vi "Get Installation Software Set.vi"(8 "error in (no error)":errorcluster, 11 "config session in":refnum<k21> caption="session in") -> (0 "error out":errorcluster, 1 "add-ons":T1[](array[typedef]) {"component type" items=["standard", "hidden", "system", "unknown", "startup"]}, 2 "software set":T1 {"component type" items=["standard", "hidden", "system", "unknown", "startup"]}, 3 "config session out":refnum<k21> caption="session out")   [LabVIEW 2013]
uses:
  <vilib>/nisyscfg/Software 1.2.ctl
  <vilib>/nisyscfg/Component Type.ctl
  <vilib>/nisyscfg/Get Available Sets.vi
  globals/Globals.vi
  <vilib>/nisyscfg/nisyscfg.lvlib
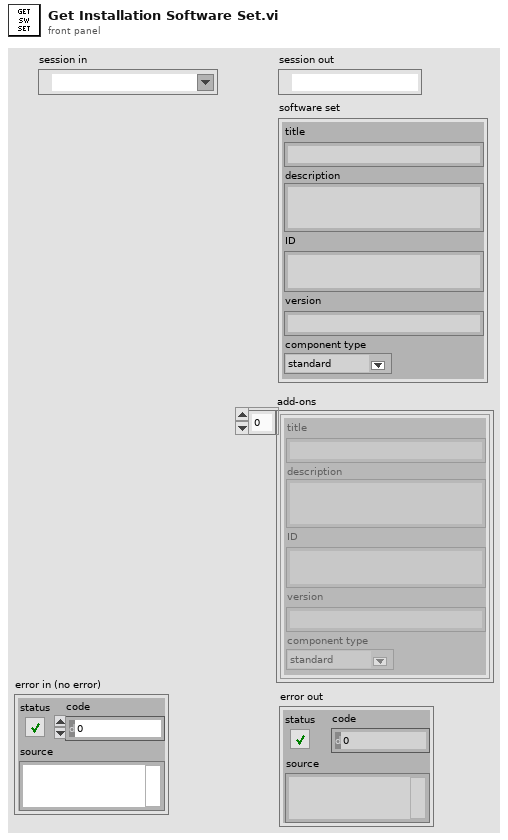
[diagram p1: front panel]
types:
  T1 = typedef "nisyscfg.lvlib/Software 1.2.ctl" = cluster{"title":string, "description":string, "ID":string, "version":string, "component type":T2}
  T2 = typedef "nisyscfg.lvlib/Component Type.ctl" = u32
  T3 = typedef "nisyscfg.lvlib/Software Set 1.2.ctl" = cluster{"information":T1, "items":T1[], "add-ons":T1[]}
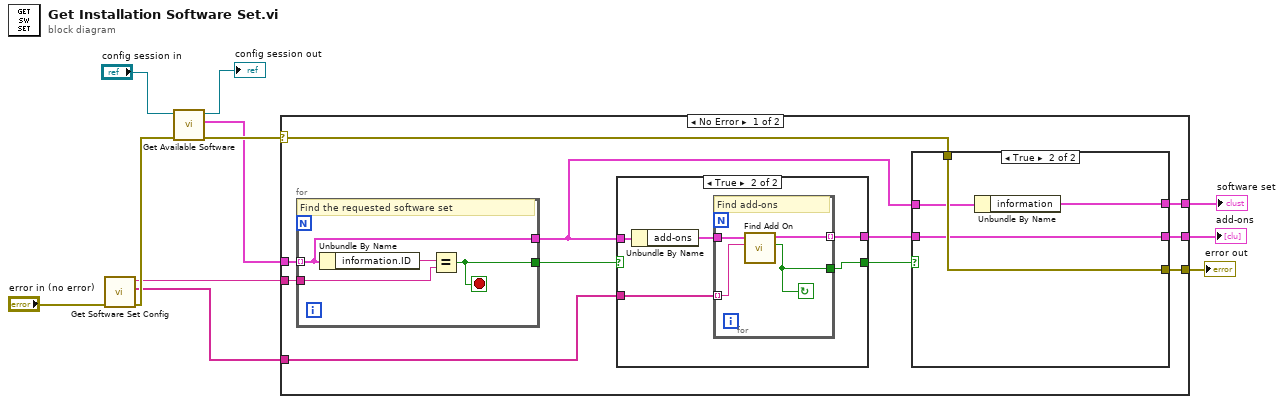
[diagram p0: block diagram]
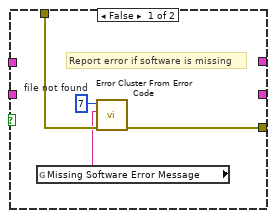
[diagram p2: hidden frame]
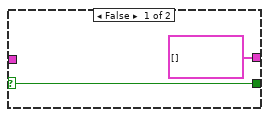
[diagram p3: hidden frame]
diagram:
  n1 = call "Get Software Set Config.vi"("error in (no error)"="error in (no error)") -> ("error out"=w8:errorcluster, "add on guids"=w4:string[], "software set guid"=w6:string)  [unwired: 8 in]
  n2 = call-poly <vilib>:"Get Available Software.vi"("error in (no error)"=w8, "session in"="config session in") -> ("error out"=w11:errorcluster, "software sets"=w7:T3[], "session out"=→"config session out":refnum<k21>)  [unwired: 7 in]
  n3 = case shown="No Error" w11 {
    selector: w11 -> [w17 w46]
    tunnel: w7 -> [w22 _]
    tunnel: w6 -> [w21 _]
    tunnel: w4 -> [w19 _]
    tunnel: [w16 w46] -> w3
    tunnel: [w13 _] -> w2
    tunnel: [w12 _] -> w1
    frame No Error {
      n4 = for {
        tunnel: w22 -> [w43] mode=indexing
        tunnel: w21 -> [w44]
        tunnel: [w43] -> w14
        tunnel: [w42] -> w20
        stop <- w42 stop-if-true
        # "Find the requested software set"
        n5 = Unbundle By Name(w43) -> ("information.ID"=w45:string)
        n6 = Equal?(x=w45, y=w44) -> (x = y?=w42:bool)
      }
      n7 = case shown="True" w20 {
        selector: w20 -> [w31 _]
        tunnel: w19 -> [_ w37]
        tunnel: w14 -> [_ w36]
        tunnel: [w31 w34] -> w18
        tunnel: [T1[] [] w33] -> w15
        frame False {
        }
        frame True {
          n8 = Unbundle By Name(w36) -> ("add-ons"=w35:T1[])
          n9 = for {
            tunnel: w37 -> [w40] mode=indexing
            tunnel: w35 -> [w41]
            tunnel: [w39] -> w33 mode=indexing
            tunnel: [w38] -> w34
            stop <- w38 continue-if-true
            # "Find add-ons"
            n10 = call "Find Add On.vi"("requested add-on guid"=w40, "add-ons"=w41) -> ("found?"=w38:bool, "add-on"=w39:T1)  [unwired: 8 in]
          }
        }
      }
      n11 = case shown="True" w18 {
        tunnel: w17 -> [w26 w30]
        tunnel: [w23 w30] -> w16
        tunnel: w15 -> [_ w28]
        tunnel: w14 -> [_ w29]
        tunnel: [_ w28] -> w13
        tunnel: [_ w27] -> w12
        frame False {
          w25 = 7  # file not found
          # "Report error if software is missing"
          n12 = global read "Globals.vi" "Missing Software Error Message"() -> (w24:string)
          n13 = call <vilib>:"Error Cluster From Error Code.vi"("error in (no error)"=w26, "error message (\"\")"=w24, "error code (0)"=w25) -> ("error out"=w23:errorcluster)  [unwired: 6 in]
        }
        frame True {
          n14 = Unbundle By Name(w29) -> ("information"=w27:T1)
        }
      }
    }
    frame Error {
    }
  }
  "error out" <- w3
  "software set" <- w1
  "add-ons" <- w2
